vi "VISJS Viewer.vi"(4 "Extra Scripts":string, 5 "FileDependency out":map{path, T1}(c390), 6 "Options":string, 7 "OpenWebBrowser(False)":bool, 8 "error in":errorcluster, 9 "Embedd VISJS Librarya in HTMl File(False)":bool, 10 "HTMLFilePath":path, 11 "LibraryDependency":map{path, T3}(c390)) -> (0 "error out":errorcluster, 3 "HTMLFileContent":string)   [LabVIEW 2020, in "VISJS Viewer.lvlib"] (continued)
  w39 = "/**\n * vis-network\n * https://visjs.github.io/vis-network/\n *\n * A dynamic, browser-based visualization library.\n *\n * @version 0.0.0-no-version\n * @date    2024-08-26T06:20:20.413Z\n *\n * @copyright (c) 2011-2017 Almende B.V, http://almende.com\n * @copyright (c) 2017-2019 visjs contributors, https://github.com/visjs\n *\n * @license\n * vis.js is dual licensed under both\n *\n *   1. The Apache 2.0 License\n *      http://www.apache.org/licenses/LICENSE-2.0\n *\n *   and\n *\n *   2. The MIT License\n *      http://opensource.org/licenses/MIT\n *\n * vis.js may be distributed under either license.\n */\n!function(g,t){\"object\"==typeof exports&&\"undefined\"!=typeof module?t(exports):\"function\"==typeof define&&define.amd?define([\"exports\"],t):t((g=\"undefined\"!=typeof globalThis?globalThis:g||self).vis=g.vis||{})}(this,(function(g){var t=\"undefined\"!=typeof globalThis?globalThis:\"undefined\"!=typeof window?window:\"undefined\"!=typeof global?global:\"undefined\"!=typeof self?self:{};function A(g){return g&&g.__esModule&&Object.prototype.hasOwnProperty.call(g,\"default\")?g.default:g}var e=function(g){return g&&g.Math===Math&&g},C=e(\"object\"==typeof globalThis&&globalThis)||e(\"object\"==typeof window&&window)||e(\"object\"==typeof self&&self)||e(\"object\"==typeof t&&t)||function(){return this}()||t||Function(\"return this\")(),I=function(g){try{return!!g()}catch(g){return!0}},i=!I((function(){var g=function(){}.bind();return\"function\"!=typeof g||g.hasOwnProperty(\"prototype\")})),o=i,n=Function.prototype,r=n.apply,s=n.call,a=\"object\"==typeof Reflect&&Reflect.apply||(o?s.bind(r):function(){return s.apply(r,arguments)}),d=i,h=Function.prototype,l=h.call,c=d&&h.bind.bind(l,l),u=d?c:function(g){return function(){return l.apply(g,arguments)}},p=u,f=p({}.toString),v=p(\"\".slice),y=function(g){return v(f(g),8,-1)},m=y,b=u,w=function(g){if(\"Function\"===m(g))return b(g)},k=\"object\"==typeof document&&document.all,x={all:k,IS_HTMLDDA:void 0===k&&void 0!==k},E=x.all,O=x.IS_HTMLDDA?function(g){return\"function\"==typeof g||g===E}:function(g){return\"function\"==typeof g},T={},D=!I((function(){return 7!==Object.defineProperty({},1,{get:function(){return 7}})[1]})),N=i,R=Function.prototype.call,P=N?R.bind(R):function(){return R.apply(R,arguments)},M={},B={}.propertyIsEnumerable,z=Object.getOwnPropertyDescriptor,S=z&&!B.call({1:2},1);M.f=S?function(g){var t=z(this,g);return!!t&&t.enumerable}:B;var Z,F,G=function(g,t){return{enumerable:!(1&g),configurable:!(2&g),writable:!(4&g),value:t}},j=I,L=y,V=Object,Y=u(\"\".split),W=j((function(){return!V(\"z\").propertyIsEnumerable(0)}))?function(g){return\"String\"===L(g)?Y(g,\"\"):V(g)}:V,Q=function(g){return null==g},U=Q,_=TypeError,K=function(g){if(U(g))throw new _(\"Can't call method on \"+g);return g},H=W,X=K,J=function(g){return H(X(g))},q=O,$=x.all,gg=x.IS_HTMLDDA?function(g){return\"object\"==typeof g?null!==g:q(g)||g===$}:function(g){return\"object\"==typeof g?null!==g:q(g)},tg={},Ag=tg,eg=C,Cg=O,Ig=function(g){return Cg(g)?g:void 0},ig=function(g,t){return arguments.length<2?Ig(Ag[g])||Ig(eg[g]):Ag[g]&&Ag[g][t]||eg[g]&&eg[g][t]},og=u({}.isPrototypeOf),ng=\"undefined\"!=typeof navigator&&String(navigator.userAgent)||\"\",rg=C,sg=ng,ag=rg.process,dg=rg.Deno,hg=ag&&ag.versions||dg&&dg.version,lg=hg&&hg.v8;lg&&(F=(Z=lg.split(\".\"))[0]>0&&Z[0]<4?1:+(Z[0]+Z[1])),!F&&sg&&(!(Z=sg.match(/Edge\\/(\\d+)/))||Z[1]>=74)&&(Z=sg.match(/Chrome\\/(\\d+)/))&&(F=+Z[1]);var cg=F,ug=cg,pg=I,fg=C.String,vg=!!Object.getOwnPropertySymbols&&!pg((function(){var g=Symbol(\"symbol detection\");return!fg(g)||!(Object(g)instanceof Symbol)||!Symbol.sham&&ug&&ug<41})),yg=vg&&!Symbol.sham&&\"symbol\"==typeof Symbol.iterator,mg=ig,bg=O,wg=og,kg=Object,xg=yg?function(g){return\"symbol\"==typeof g}:function(g){var t=mg(\"Symbol\");return bg(t)&&wg(t.prototype,kg(g))},Eg=String,Og=function(g){try{return Eg(g)}catch(g){return\"Object\"}},Tg=O,Dg=Og,Ng=TypeError,Rg=function(g){if(Tg(g))return g;throw new Ng(Dg(g)+\" is not a function\")},Pg=Rg,Mg=Q,Bg=function(g,t){var A=g[t];return Mg(A)?void 0:Pg(A)},zg=P,Sg=O,Zg=gg,Fg=TypeError,Gg={exports:{}},jg=C,Lg=Object.defineProperty,Vg=function(g,t){try{Lg(jg,g,{value:t,configurable:!0,writable:!0})}catch(A){jg[g]=t}return t},Yg=\"__core-js_shared__\",Wg=C[Yg]||Vg(Yg,{}),Qg=Wg;(Gg.exports=function(g,t){return Qg[g]||(Qg[g]=void 0!==t?t:{})})(\"versions\",[]).push({version:\"3.33.0\",mode:\"pure\",copyright:\"© 2014-2023 Denis Pushkarev (zloirock.ru)\",license:\"https://github.com/zloirock/core-js/blob/v3.33.0/LICENSE\",source:\"https://github.com/zloirock/core-js\"});var Ug=Gg.exports,_g=K,Kg=Object,Hg=function(g){return Kg(_g(g))},Xg=Hg,Jg=u({}.hasOwnProperty),qg=Object.hasOwn||function(g,t){return Jg(Xg(g),t)},$g=u,gt=0,tt=Math.random(),At=$g(1..toString),et=function(g){return\"Symbol(\"+(void 0===g?\"\":g)+\")_\"+At(++gt+tt,36)},Ct=Ug,It=qg,it=et,ot=vg,nt=yg,rt=C.Symbol,st=Ct(\"wks\"),at=nt?rt.for||rt:rt&&rt.withoutSetter||it,dt=function(g){return It(st,g)||(st[g]=ot&&It(rt,g)?rt[g]:at(\"Symbol.\"+g)),st[g]},ht=P,lt=gg,ct=xg,ut=Bg,pt=function(g,t){var A,e;if(\"string\"===t&&Sg(A=g.toString)&&!Zg(e=zg(A,g)))return e;if(Sg(A=g.valueOf)&&!Zg(e=zg(A,g)))return e;if(\"string\"!==t&&Sg(A=g.toString)&&!Zg(e=zg(A,g)))return e;throw new Fg(\"Can't convert object to primitive value\")},ft=TypeError,vt=dt(\"toPrimitive\"),yt=function(g,t){if(!lt(g)||ct(g))return g;var A,e=ut(g,vt);if(e){if(void 0===t&&(t=\"default\"),A=ht(e,g,t),!lt(A)||ct(A))return A;throw new ft(\"Can't convert object to primitive value\")}return void 0===t&&(t=\"number\"),pt(g,t)},mt=xg,bt=function(g){var t=yt(g,\"string\");return mt(t)?t:t+\"\"},wt=gg,kt=C.document,xt=wt(kt)&&wt(kt.createElement),Et=function(g){return xt?kt.createElement(g):{}},Ot=Et,Tt=!D&&!I((function(){return 7!==Object.defineProperty(Ot(\"div\"),\"a\",{get:function(){return 7}}).a})),Dt=D,Nt=P,Rt=M,Pt=G,Mt=J,Bt=bt,zt=qg,St=Tt,Zt=Object.getOwnPropertyDescriptor;T.f=Dt?Zt:function(g,t){if(g=Mt(g),t=Bt(t),St)try{return Zt(g,t)}catch(g){}if(zt(g,t))return Pt(!Nt(Rt.f,g,t),g[t])};var Ft=I,Gt=O,jt=/#|\\.prototype\\./,Lt=function(g,t){var A=Yt[Vt(g)];return A===Qt||A!==Wt&&(Gt(t)?Ft(t):!!t)},Vt=Lt.normalize=function(g){return String(g).replace(jt,\".\").toLowerCase()},Yt=Lt.data={},Wt=Lt.NATIVE=\"N\",Qt=Lt.POLYFILL=\"P\",Ut=Lt,_t=Rg,Kt=i,Ht=w(w.bind),Xt=function(g,t){return _t(g),void 0===t?g:Kt?Ht(g,t):function(){return g.apply(t,arguments)}},Jt={},qt=D&&I((function(){return 42!==Object.defineProperty((function(){}),\"prototype\",{value:42,writable:!1}).prototype})),$t=gg,gA=String,tA=TypeError,AA=function(g){if($t(g))return g;throw new tA(gA(g)+\" is not an object\")},eA=D,CA=Tt,IA=qt,iA=AA,oA=bt,nA=TypeError,rA=Object.defineProperty,sA=Object.getOwnPropertyDescriptor,aA=\"enumerable\",dA=\"configurable\",hA=\"writable\";Jt.f=eA?IA?function(g,t,A){if(iA(g),t=oA(t),iA(A),\"function\"==typeof g&&\"prototype\"===t&&\"value\"in A&&hA in A&&!A[hA]){var e=sA(g,t);e&&e[hA]&&(g[t]=A.value,A={configurable:dA in A?A[dA]:e[dA],enumerable:aA in A?A[aA]:e[aA],writable:!1})}return rA(g,t,A)}:rA:function(g,t,A){if(iA(g),t=oA(t),iA(A),CA)try{return rA(g,t,A)}catch(g){}if(\"get\"in A||\"set\"in A)throw new nA(\"Accessors not supported\");return\"value\"in A&&(g[t]=A.value),g};var lA=Jt,cA=G,uA=D?function(g,t,A){return lA.f(g,t,cA(1,A))}:function(g,t,A){return g[t]=A,g},pA=C,fA=a,vA=w,yA=O,mA=T.f,bA=Ut,wA=tg,kA=Xt,xA=uA,EA=qg,OA=function(g){var t=function(A,e,C){if(this instanceof t){switch(arguments.length){case 0:return new g;case 1:return new g(A);case 2:return new g(A,e)}return new g(A,e,C)}return fA(g,this,arguments)};return t.prototype=g.prototype,t},TA=function(g,t){var A,e,C,I,i,o,n,r,s,a=g.target,d=g.global,h=g.stat,l=g.proto,c=d?pA:h?pA[a]:(pA[a]||{}).prototype,u=d?wA:wA[a]||xA(wA,a,{})[a],p=u.prototype;for(I in t)e=!(A=bA(d?I:a+(h?\".\":\"#\")+I,g.forced))&&c&&EA(c,I),o=u[I],e&&(n=g.dontCallGetSet?(s=mA(c,I))&&s.value:c[I]),i=e&&n?n:t[I],e&&typeof o==typeof i||(r=g.bind&&e?kA(i,pA):g.wrap&&e?OA(i):l&&yA(i)?vA(i):i,(g.sham||i&&i.sham||o&&o.sham)&&xA(r,\"sham\",!0),xA(u,I,r),l&&(EA(wA,C=a+\"Prototype\")||xA(wA,C,{}),xA(wA[C],I,i),g.real&&p&&(A||!p[I])&&xA(p,I,i)))},DA=Math.ceil,NA=Math.floor,RA=Math.trunc||function(g){var t=+g;return(t>0?NA:DA)(t)},PA=function(g){var t=+g;return t!=t||0===t?0:RA(t)},MA=PA,BA=Math.max,zA=Math.min,SA=function(g,t){var A=MA(g);return A<0?BA(A+t,0):zA(A,t)},ZA=PA,FA=Math.min,GA=function(g){return g>0?FA(ZA(g),9007199254740991):0},jA=function(g){return GA(g.length)},LA=J,VA=SA,YA=jA,WA=function(g){return function(t,A,e){var C,I=LA(t),i=YA(I),o=VA(e,i);if(g&&A!=A){for(;i>o;)if((C=I[o++])!=C)return!0}else for(;i>o;o++)if((g||o in I)&&I[o]===A)return g||o||0;return!g&&-1}},QA={includes:WA(!0),indexOf:WA(!1)},UA={},_A=qg,KA=J,HA=QA.indexOf,XA=UA,JA=u([].push),qA=function(g,t){var A,e=KA(g),C=0,I=[];for(A in e)!_A(XA,A)&&_A(e,A)&&JA(I,A);for(;t.length>C;)_A(e,A=t[C++])&&(~HA(I,A)||JA(I,A));return I},$A=[\"constructor\",\"hasOwnProperty\",\"isPrototypeOf\",\"propertyIsEnumerable\",\"toLocaleString\",\"toString\",\"valueOf\"],ge=qA,te=$A,Ae=Object.keys||function(g){return ge(g,te)},ee={};ee.f=Object.getOwnPropertySymbols;var Ce=D,Ie=u,ie=P,oe=I,ne=Ae,re=ee,se=M,ae=Hg,de=W,he=Object.assign,le=Object.defineProperty,ce=Ie([].concat),ue=!he||oe((function(){if(Ce&&1!==he({b:1},he(le({},\"a\",{enumerable:!0,get:function(){le(this,\"b\",{value:3,enumerable:!1})}}),{b:2})).b)return!0;var g={},t={},A=Symbol(\"assign detection\"),e=\"abcdefghijklmnopqrst\";return g[A]=7,e.split(\"\").forEach((function(g){t[g]=g})),7!==he({},g)[A]||ne(he({},t)).join(\"\")!==e}))?function(g,t){for(var A=ae(g),e=arguments.length,C=1,I=re.f,i=se.f;e>C;)for(var o,n=de(arguments[C++]),r=I?ce(ne(n),I(n)):ne(n),s=r.length,a=0;s>a;)o=r[a++],Ce&&!ie(i,n,o)||(A[o]=n[o]);return A}:he,pe=ue;TA({target:\"Object\",stat:!0,arity:2,forced:Object.assign!==pe},{assign:pe});var fe=A(tg.Object.assign),ve=u([].slice),ye=u,me=Rg,be=gg,we=qg,ke=ve,xe=i,Ee=Function,Oe=ye([].concat),Te=ye([].join),De={},Ne=xe?Ee.bind:function(g){var t=me(this),A=t.prototype,e=ke(arguments,1),C=function(){var A=Oe(e,ke(arguments));return this instanceof C?function(g,t,A){if(!we(De,t)){for(var e=[],C=0;C<t;C++)e[C]=\"a[\"+C+\"]\";De[t]=Ee(\"C,a\",\"return new C(\"+Te(e,\",\")+\")\")}return De[t](g,A)}(t,A.length,A):t.apply(g,A)};return be(A)&&(C.prototype=A),C},Re=Ne;TA({target:\"Function\",proto:!0,forced:Function.bind!==Re},{bind:Re});var Pe=tg,Me=function(g){return Pe[g+\"Prototype\"]},Be=Me(\"Function\").bind,ze=og,Se=Be,Ze=Function.prototype,Fe=function(g){var t=g.bind;return g===Ze||ze(Ze,g)&&t===Ze.bind?Se:t},Ge=Fe,je=A(Ge);function Le(g,t,A,e){g.beginPath(),g.arc(t,A,e,0,2*Math.PI,!1),g.closePath()}function Ve(g,t,A,e,C,I){var i=Math.PI/180;e-2*I<0&&(I=e/2),C-2*I<0&&(I=C/2),g.beginPath(),g.moveTo(t+I,A),g.lineTo(t+e-I,A),g.arc(t+e-I,A+I,I,270*i,360*i,!1),g.lineTo(t+e,A+C-I),g.arc(t+e-I,A+C-I,I,0,90*i,!1),g.lineTo(t+I,A+C),g.arc(t+I,A+C-I,I,90*i,180*i,!1),g.lineTo(t,A+I),g.arc(t+I,A+I,I,180*i,270*i,!1),g.closePath()}function Ye(g,t,A,e,C){var I=.5522848,i=e/2*I,o=C/2*I,n=t+e,r=A+C,s=t+e/2,a=A+C/2;g.beginPath(),g.moveTo(t,a),g.bezierCurveTo(t,a-o,s-i,A,s,A),g.bezierCurveTo(s+i,A,n,a-o,n,a),g.bezierCurveTo(n,a+o,s+i,r,s,r),g.bezierCurveTo(s-i,r,t,a+o,t,a),g.closePath()}function We(g,t,A,e,C){var I=C*(1/3),i=.5522848,o=e/2*i,n=I/2*i,r=t+e,s=A+I,a=t+e/2,d=A+I/2,h=A+(C-I/2),l=A+C;g.beginPath(),g.moveTo(r,d),g.bezierCurveTo(r,d+n,a+o,s,a,s),g.bezierCurveTo(a-o,s,t,d+n,t,d),g.bezierCurveTo(t,d-n,a-o,A,a,A),g.bezierCurveTo(a+o,A,r,d-n,r,d),g.lineTo(r,h),g.bezierCurveTo(r,h+n,a+o,l,a,l),g.bezierCurveTo(a-o,l,t,h+n,t,h),g.lineTo(t,d)}function Qe(g,t,A,e,C,I){g.beginPath(),g.moveTo(t,A);for(var i=I.length,o=e-t,n=C-A,r=n/o,s=Math.sqrt(o*o+n*n),a=0,d=!0,h=0,l=+I[0];s>=.1;)(l=+I[a++%i])>s&&(l=s),h=Math.sqrt(l*l/(1+r*r)),t+=h=o<0?-h:h,A+=r*h,!0===d?g.lineTo(t,A):g.moveTo(t,A),s-=l,d=!d}var Ue={circle:Le,dashedLine:Qe,database:We,diamond:function(g,t,A,e){g.beginPath(),g.lineTo(t,A+e),g.lineTo(t+e,A),g.lineTo(t,A-e),g.lineTo(t-e,A),g.closePath()},ellipse:Ye,ellipse_vis:Ye,hexagon:function(g,t,A,e){g.beginPath();var C=2*Math.PI/6;g.moveTo(t+e,A);for(var I=1;I<6;I++)g.lineTo(t+e*Math.cos(C*I),A+e*Math.sin(C*I));g.closePath()},roundRect:Ve,square:function(g,t,A,e){g.beginPath(),g.rect(t-e,A-e,2*e,2*e),g.closePath()},star:function(g,t,A,e){g.beginPath(),A+=.1*(e*=.82);for(var C=0;C<10;C++){var I=C%2==0?1.3*e:.5*e;g.lineTo(t+I*Math.sin(2*C*Math.PI/10),A-I*Math.cos(2*C*Math.PI/10))}g.closePath()},triangle:function(g,t,A,e){g.beginPath(),A+=.275*(e*=1.15);var C=2*e,I=C/2,i=Math.sqrt(3)/6*C,o=Math.sqrt(C*C-I*I);g.moveTo(t,A-(o-i)),g.lineTo(t+I,A+i),g.lineTo(t-I,A+i),g.lineTo(t,A-(o-i)),g.closePath()},triangleDown:function(g,t,A,e){g.beginPath(),A-=.275*(e*=1.15);var C=2*e,I=C/2,i=Math.sqrt(3)/6*C,o=Math.sqrt(C*C-I*I);g.moveTo(t,A+(o-i)),g.lineTo(t+I,A-i),g.lineTo(t-I,A-i),g.lineTo(t,A+(o-i)),g.closePath()}};function _e(g,t){void 0===t&&(t={});var A=t.insertAt;if(g&&\"undefined\"!=typeof document){var e=document.head||document.getElementsByTagName(\"head\")[0],C=document.createElement(\"style\");C.type=\"text/css\",\"top\"===A&&e.firstChild?e.insertBefore(C,e.firstChild):e.appendChild(C),C.styleSheet?C.styleSheet.cssText=g:C.appendChild(document.createTextNode(g))}}_e(\".vis-overlay{bottom:0;left:0;position:absolute;right:0;top:0;z-index:10}.vis-active{box-shadow:0 0 10px #86d5f8}\");_e(\".vis [class*=span]{min-height:0;width:auto}\");_e('div.vis-color-picker{background-color:#fff;border-radius:15px;box-shadow:0 0 10px 0 rgba(0,0,0,.5);display:none;height:444px;left:30px;margin-left:30px;margin-top:-140px;padding:10px;position:absolute;top:0;width:310px;z-index:1}div.vis-color-picker div.vis-arrow{left:5px;position:absolute;top:147px}div.vis-color-picker div.vis-arrow:after,div.vis-color-picker div.vis-arrow:before{border:solid transparent;content:\" \";height:0;pointer-events:none;position:absolute;right:100%;top:50%;width:0}div.vis-color-picker div.vis-arrow:after{border-color:hsla(0,0%,100%,0) #fff hsla(0,0%,100%,0) hsla(0,0%,100%,0);border-width:30px;margin-top:-30px}div.vis-color-picker div.vis-color{cursor:pointer;height:289px;position:absolute;width:289px}div.vis-color-picker div.vis-brightness{position:absolute;top:313px}div.vis-color-picker div.vis-opacity{position:absolute;top:350px}div.vis-color-picker div.vis-selector{background:#4c4c4c;background:-moz-linear-gradient(top,#4c4c4c 0,#595959 12%,#666 25%,#474747 39%,#2c2c2c 50%,#000 51%,#111 60%,#2b2b2b 76%,#1c1c1c 91%,#131313 100%);background:-webkit-gradient(linear,left top,left bottom,color-stop(0,#4c4c4c),color-stop(12%,#595959),color-stop(25%,#666),color-stop(39%,#474747),color-stop(50%,#2c2c2c),color-stop(51%,#000),color-stop(60%,#111),color-stop(76%,#2b2b2b),color-stop(91%,#1c1c1c),color-stop(100%,#131313));background:-webkit-linear-gradient(top,#4c4c4c,#595959 12%,#666 25%,#474747 39%,#2c2c2c 50%,#000 51%,#111 60%,#2b2b2b 76%,#1c1c1c 91%,#131313);background:-o-linear-gradient(top,#4c4c4c 0,#595959 12%,#666 25%,#474747 39%,#2c2c2c 50%,#000 51%,#111 60%,#2b2b2b 76%,#1c1c1c 91%,#131313 100%);background:-ms-linear-gradient(top,#4c4c4c 0,#595959 12%,#666 25%,#474747 39%,#2c2c2c 50%,#000 51%,#111 60%,#2b2b2b 76%,#1c1c1c 91%,#131313 100%);background:linear-gradient(180deg,#4c4c4c 0,#595959 12%,#666 25%,#474747 39%,#2c2c2c 50%,#000 51%,#111 60%,#2b2b2b 76%,#1c1c1c 91%,#131313);border:1px solid #fff;border-radius:15px;filter:progid:DXImageTransform.Microsoft.gradient(startColorstr=\"#4c4c4c\",endColorstr=\"#131313\",GradientType=0);height:15px;left:137px;position:absolute;top:137px;width:15px}div.vis-color-picker div.vis-new-color{left:159px;padding-right:2px;text-align:right}div.vis-color-picker div.vis-initial-color,div.vis-color-picker div.vis-new-color{border:1px solid rgba(0,0,0,.1);border-radius:5px;color:rgba(0,0,0,.4);font-size:10px;height:20px;line-height:20px;position:absolute;top:380px;vertical-align:middle;width:140px}div.vis-color-picker div.vis-initial-color{left:10px;padding-left:2px;text-align:left}div.vis-color-picker div.vis-label{left:10px;position:absolute;width:300px}div.vis-color-picker div.vis-label.vis-brightness{top:300px}div.vis-color-picker div.vis-label.vis-opacity{top:338px}div.vis-color-picker div.vis-button{background-color:#f7f7f7;border:2px solid #d9d9d9;border-radius:10px;cursor:pointer;height:25px;line-height:25px;position:absolute;text-align:center;top:410px;vertical-align:middle;width:68px}div.vis-color-picker div.vis-button.vis-cancel{left:5px}div.vis-color-picker div.vis-button.vis-load{left:82px}div.vis-color-picker div.vis-button.vis-apply{left:159px}div.vis-color-picker div.vis-button.vis-save{left:236px}div.vis-color-picker input.vis-range{height:20px;width:290px}');_e('div.vis-configuration{display:block;float:left;font-size:12px;position:relative}div.vis-configuration-wrapper{display:block;width:700px}div.vis-configuration-wrapper:after{clear:both;content:\"\";display:block}div.vis-configuration.vis-config-option-container{background-color:#fff;border:2px solid #f7f8fa;border-radius:4px;display:block;left:10px;margin-top:20px;padding-left:5px;width:495px}div.vis-configuration.vis-config-button{background-color:#f7f8fa;border:2px solid #ceced0;border-radius:4px;cursor:pointer;display:block;height:25px;left:10px;line-height:25px;margin-bottom:30px;margin-top:20px;padding-left:5px;vertical-align:middle;width:495px}div.vis-configuration.vis-config-button.hover{background-color:#4588e6;border:2px solid #214373;color:#fff}div.vis-configuration.vis-config-item{display:block;float:left;height:25px;line-height:25px;vertical-align:middle;width:495px}div.vis-configuration.vis-config-item.vis-config-s2{background-color:#f7f8fa;border-radius:3px;left:10px;padding-left:5px}div.vis-configuration.vis-config-item.vis-config-s3{background-color:#e4e9f0;border-radius:3px;left:20px;padding-left:5px}div.vis-configuration.vis-config-item.vis-config-s4{background-color:#cfd8e6;border-radius:3px;left:30px;padding-left:5px}div.vis-configuration.vis-config-header{font-size:18px;font-weight:700}div.vis-configuration.vis-config-label{height:25px;line-height:25px;width:120px}div.vis-configuration.vis-config-label.vis-config-s3{width:110px}div.vis-configuration.vis-config-label.vis-config-s4{width:100px}div.vis-configuration.vis-config-colorBlock{border:1px solid #444;border-radius:2px;cursor:pointer;height:19px;margin:0;padding:0;top:1px;width:30px}input.vis-configuration.vis-config-checkbox{left:-5px}input.vis-configuration.vis-config-rangeinput{margin:0;padding:1px;pointer-events:none;position:relative;top:-5px;width:60px}input.vis-configuration.vis-config-range{-webkit-appearance:none;background-color:transparent;border:0 solid #fff;height:20px;width:300px}input.vis-configuration.vis-config-range::-webkit-slider-runnable-track{background:#dedede;background:-moz-linear-gradient(top,#dedede 0,#c8c8c8 99%);background:-webkit-gradient(linear,left top,left bottom,color-stop(0,#dedede),color-stop(99%,#c8c8c8));background:-webkit-linear-gradient(top,#dedede,#c8c8c8 99%);background:-o-linear-gradient(top,#dedede 0,#c8c8c8 99%);background:-ms-linear-gradient(top,#dedede 0,#c8c8c8 99%);background:linear-gradient(180deg,#dedede 0,#c8c8c8 99%);border:1px solid #999;border-radius:3px;box-shadow:0 0 3px 0 #aaa;filter:progid:DXImageTransform.Microsoft.gradient(startColorstr=\"#dedede\",endColorstr=\"#c8c8c8\",GradientType=0);height:5px;width:300px}input.vis-configuration.vis-config-range::-webkit-slider-thumb{-webkit-appearance:none;background:#3876c2;background:-moz-linear-gradient(top,#3876c2 0,#385380 100%);background:-webkit-gradient(linear,left top,left bottom,color-stop(0,#3876c2),color-stop(100%,#385380));background:-webkit-linear-gradient(top,#3876c2,#385380);background:-o-linear-gradient(top,#3876c2 0,#385380 100%);background:-ms-linear-gradient(top,#3876c2 0,#385380 100%);background:linear-gradient(180deg,#3876c2 
